vi "Configure NF Monitor Spectrum.vi"(0 "VISA resource name":refnum<visa-resource-name>, 1 "Sweep Time (0)":dbl format="%^#_6g", 2 "Enable Internal Preamp (Enabled)":bool=TRUE, 5 "Averaging Count (0)":dbl format="%^#_6g", 7 "Averaging Method (0: Exponential)":i32(ring) items=["Exponential", "Repeat"], 9 "Detection Type (0: Normal)":i32(ring) items=["Normal", "Positive Peak", "Negative Peak", "Average"], 11 "error in (no error)":errorcluster, 12 "Auto RF Port Input Attenuation (Enabled)":bool=TRUE, 13 "Manual RF Port Input Attenuation (5 dB)":dbl=5.0 format="%^#_6g") -> (4 "VISA resource name out":refnum<visa-resource-name>, 15 "error out":errorcluster)   [LabVIEW 2014, in "Agilent ESA PSA Series.lvlib"]
doc: "Configures the Monitor Spectrum measurement of the Noise Figure personality.\n\n<B>Note:</B> \n\nThis VI is only valid in Noise Figure personality. Use <B>Switch Personality</B> VI to switch to Noise Figure before calling this VI."
uses:
  Agilent ESA PSA Series.lvlib
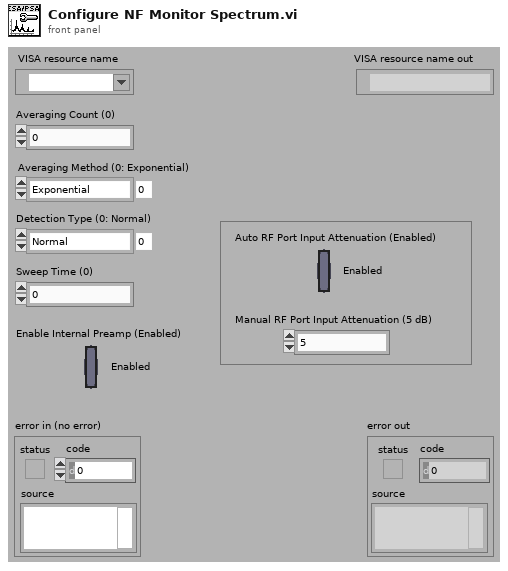
[diagram p1: front panel]
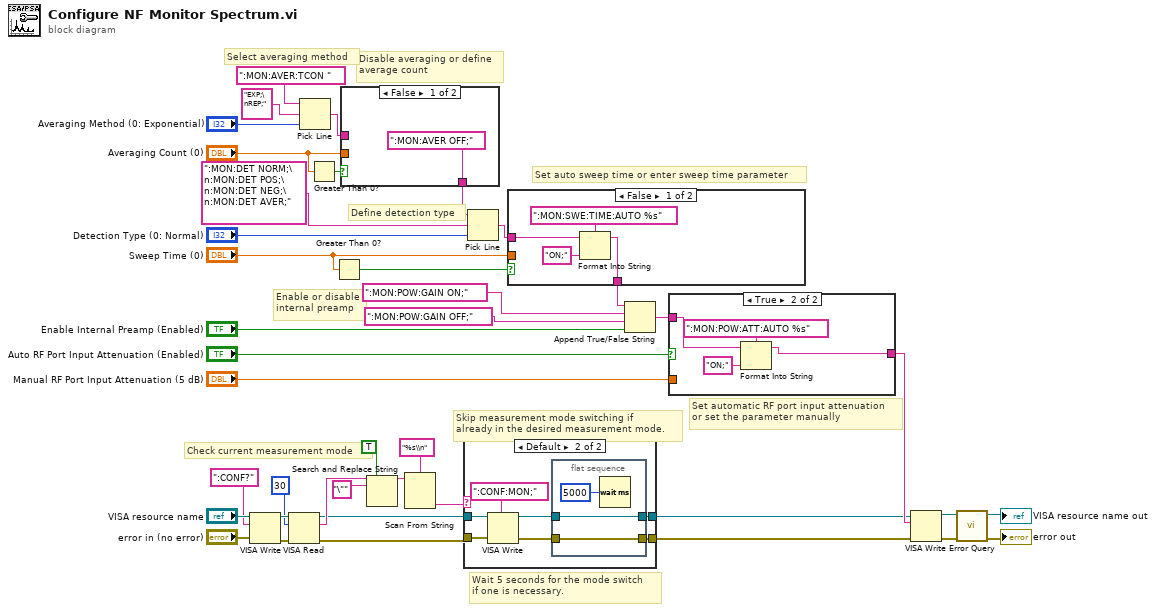
[diagram p0: block diagram]
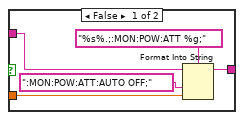
[diagram p3: hidden frame]
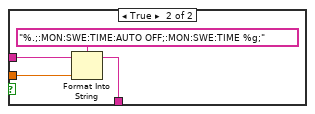
[diagram p4: hidden frame]
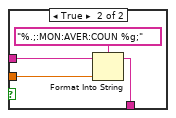
[diagram p5: hidden frame]
diagram:
  # "Enable or disable\ninternal preamp"
  # "Wait 5 seconds for the mode switch\nif one is necessary."
  # "Set automatic RF port input attenuation\nor set the parameter manually"
  # "Set auto sweep time or enter sweep time parameter"
  # "Define detection type"
  # "Disable averaging or define\naverage count"
  # "Select averaging method"
  # "Skip measurement mode switching if\nalready in the desired measurement mode."
  # "Check current measurement mode"
  n1 = VISA Write(VISA resource name="VISA resource name", write buffer=":CONF?", error in (no error)="error in (no error)") -> (VISA resource name out=w10:refnum<visa-resource-name>, error out=w11:errorcluster)  [unwired: 1 out]
  n2 = VISA Read(VISA resource name=w10, byte count=u32 30, error in (no error)=w11) -> (VISA resource name out=w2:refnum<visa-resource-name>, read buffer=w3:string, error out=w1:errorcluster)  [unwired: 1 out]
  n3 = Pick Line(string ("")=":MON:AVER:TCON ", multi-line string="EXP;\nREP;", line index="Averaging Method (0: Exponential)") -> (output string=w32:string)
  n4 = Greater Than 0?(x="Averaging Count (0)") -> (x > 0?=w31:bool)
  n5 = Greater Than 0?(x="Sweep Time (0)") -> (x > 0?=w25:bool)
  n6 = case shown="False" w31 {
    tunnel: w32 -> [_ w45]
    tunnel: "Averaging Count (0)" -> [_ w44]
    tunnel: [":MON:AVER OFF;" w42] -> w28
    frame False {
    }
    frame True {
      n7 = Format Into String(format string="%.;:MON:AVER:COUN %g;", initial string=w45, w44) -> (resulting string=w42:string)  [unwired: 1 in, 1 out]
    }
  }
  n8 = Search and Replace String(replace all?=TRUE ("replace all? (F)"), input string=w3, search string="\"") -> (result string=w6:string)  [unwired: 5 in, 3 out]
  n9 = Scan From String(format string="%s\\n", input string=w6) -> (output 1=w4:string)  [unwired: 3 in, 3 out]
  n10 = case shown="Default" w4 {
    tunnel: w2 -> [w47 w54]
    tunnel: w1 -> [w46 w53]
    tunnel: [w47 w49] -> w16
    tunnel: [w46 w48] -> w15
    frame "MON", "MONitor" {
    }
    frame Default {
      n11 = VISA Write(VISA resource name=w54, write buffer=":CONF:MON;", error in (no error)=w53) -> (VISA resource name out=w51:refnum<visa-resource-name>, error out=w50:errorcluster)  [unwired: 1 out]
      n12 = flat-sequence {
        tunnel: w51 -> [w57]
        tunnel: w50 -> [w56]
        tunnel: [w57] -> w49
        tunnel: [w56] -> w48
        frame #0 {
          n13 = Wait (ms)(milliseconds to wait=u32 5000) -> ()  [unwired: 1 out]
        }
      }
    }
  }
  n14 = Pick Line(string ("")=w28, multi-line string=":MON:DET NORM;\n:MON:DET POS;\n:MON:DET NEG;\n:MON:DET AVER;", line index="Detection Type (0: Normal)") -> (output string=w26:string)
  n15 = case shown="False" w25 {
    tunnel: [w61 w64] -> w24
    tunnel: "Sweep Time (0)" -> [_ w63]
    tunnel: w26 -> [w59 w62]
    frame False {
      n16 = Format Into String(format string=":MON:SWE:TIME:AUTO %s", initial string=w59, "ON;" ("input 1")) -> (resulting string=w61:string)  [unwired: 1 in, 1 out]
    }
    frame True {
      n17 = Format Into String(format string="%.;:MON:SWE:TIME:AUTO OFF;:MON:SWE:TIME %g;", initial string=w62, w63) -> (resulting string=w64:string)  [unwired: 1 in, 1 out]
    }
  }
  n18 = Append True/False String(1:"Enable Internal Preamp (Enabled)", 2:":MON:POW:GAIN OFF;" ("false string"), 3:":MON:POW:GAIN ON;" ("true string"), 4:w24) -> (0:w20:string)
  n19 = case shown="True" "Auto RF Port Input Attenuation (Enabled)" {
    tunnel: w20 -> [w68 w74]
    tunnel: "Manual RF Port Input Attenuation (5 dB)" -> [w70 _]
    tunnel: [w66 w71] -> w17
    frame False {
      n20 = Format Into String(format string="%s%.;:MON:POW:ATT %g;", initial string=w68, ":MON:POW:ATT:AUTO OFF;" ("format string"), w70) -> (resulting string=w66:string)  [unwired: 1 in, 1 out]
    }
    frame True {
      n21 = Format Into String(format string=":MON:POW:ATT:AUTO %s", initial string=w74, "ON;" ("input 1")) -> (resulting string=w71:string)  [unwired: 1 in, 1 out]
    }
  }
  n22 = VISA Write(VISA resource name=w16, write buffer=w17, error in (no error)=w15) -> (VISA resource name out=w38:refnum<visa-resource-name>, error out=w37:errorcluster)  [unwired: 1 out]
  n23 = call "Error Query.vi"("error in (no error)"=w37, "VISA resource name"=w38) -> ("error out"=→"error out":errorcluster, "VISA resource name out"=→"VISA resource name out":refnum<visa-resource-name>)  [unwired: 6 in, 2 out]
